vi "get_TLC_index.vi"(8 "error in (no error)":errorcluster, 11 "GenericToplevelComponent in":refnum<class "GenericToplevelComponent.lvclass">) -> (0 "error out":errorcluster, 2 "index":i32, 3 "GenericToplevelComponent out":refnum<class "GenericToplevelComponent.lvclass">)   [LabVIEW 2010, in "GenericToplevelComponent.lvclass"]
uses:
  GenericToplevelComponent.lvclass
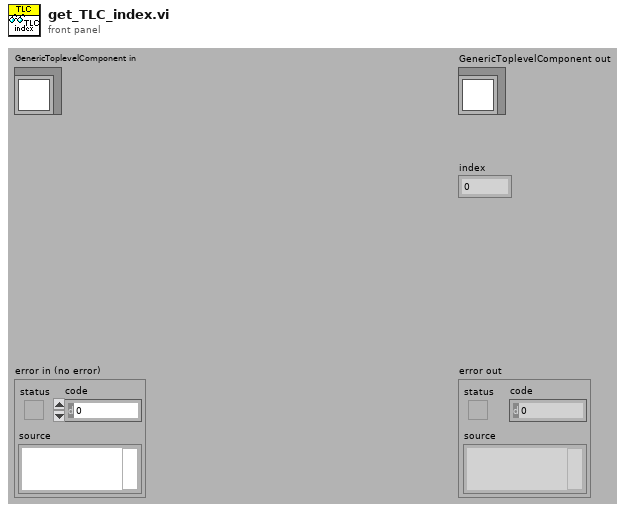
[diagram p1: front panel]
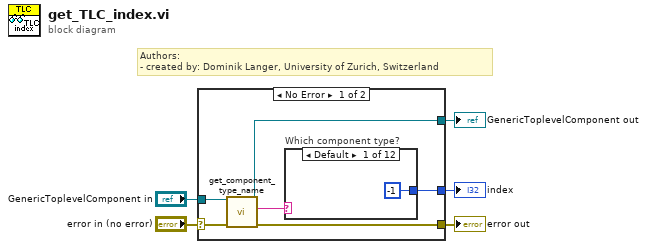
[diagram p0: block diagram]
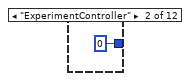
[diagram p2: hidden frame]
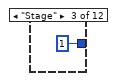
[diagram p3: hidden frame]
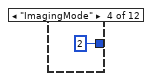
[diagram p4: hidden frame]
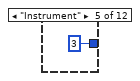
[diagram p5: hidden frame]
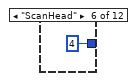
[diagram p6: hidden frame]
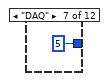
[diagram p7: hidden frame]
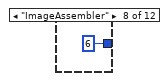
[diagram p8: hidden frame]
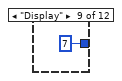
[diagram p9: hidden frame]
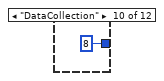
[diagram p10: hidden frame]
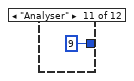
[diagram p11: hidden frame]
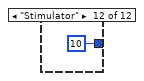
[diagram p12: hidden frame]
diagram:
  # "Authors: \n- created by: Dominik Langer, University of Zurich, Switzerland"
  n1 = case shown="No Error" "error in (no error)" {
    selector: "error in (no error)" -> [w11 w25]
    tunnel: [w10 w25] -> w4
    tunnel: [w8 w24] -> w2
    tunnel: "GenericToplevelComponent in" -> [w9 w24]
    tunnel: [w6 _] -> w1
    frame No Error {
      n2 = call-dynamic "get_component_type_name.vi"("error in (no error)"=w11, "GenericPlugin in"=w9) -> ("error out"=w10:errorcluster, "component type"=w7:string, "GenericPlugin out"=w8:refnum<class "GenericToplevelComponent.lvclass">)  [unwired: 7 in]
      n3 = case "Which component type?" shown="Default" w7 {
        tunnel: [-1 0 1 2 3 4 5 6 7 8 9 10] -> w6
        frame Default {
        }
        frame "ExperimentController" {
        }
        frame "Stage" {
        }
        frame "ImagingMode" {
        }
        frame "Instrument" {
        }
        frame "ScanHead" {
        }
        frame "DAQ" {
        }
        frame "ImageAssembler" {
        }
        frame "Display" {
        }
        frame "DataCollection" {
        }
        frame "Analyser" {
        }
        frame "Stimulator" {
        }
      }
    }
    frame Error {
    }
  }
  "error out" <- w4
  "GenericToplevelComponent out" <- w2
  "index" <- w1
